vi "GearIntakeOpen.vi"(7 "Gear Intake.lvclass":refnum<class "Gear Intake.lvclass">, 11 "Motor Refnum":string) -> (3 "Gear Intake.lvclass":refnum<class "Gear Intake.lvclass">)   [LabVIEW 2016, in "Gear Intake.lvclass"]
uses:
  Gear Intake.lvclass
  Gear Intake.lvclass/Gear Intake.ctl
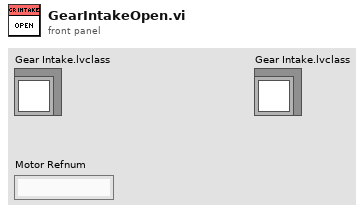
[diagram p1: front panel]
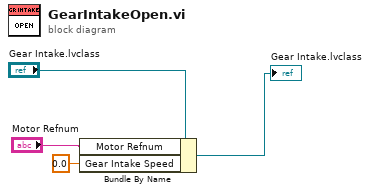
[diagram p0: block diagram]
diagram:
  n1 = Bundle By Name(cluster="Gear Intake.lvclass", "Motor Refnum"="Motor Refnum", "Gear Intake Speed"=0.0) -> (→"Gear Intake.lvclass":refnum<class "Gear Intake.lvclass">)
